vi "Get Devices List.vi"(0 "SLSC Interface in":refnum<class "SLSC Interface.lvclass">, 11 "error in (no error)":errorcluster) -> (4 "SLSC Interface out":refnum<class "SLSC Interface.lvclass">, 8 "Sys.Devices":refnum<k21>[](array[refnum]), 15 "error out":errorcluster)   [LabVIEW 2015, in "SLSC Interface.lvclass"]
uses:
  SLSC Interface.lvclass
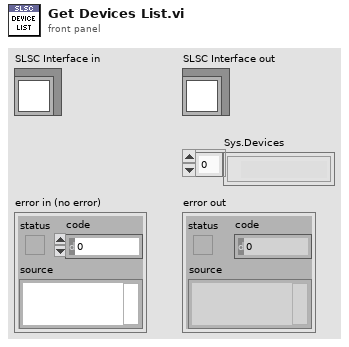
[diagram p1: front panel]
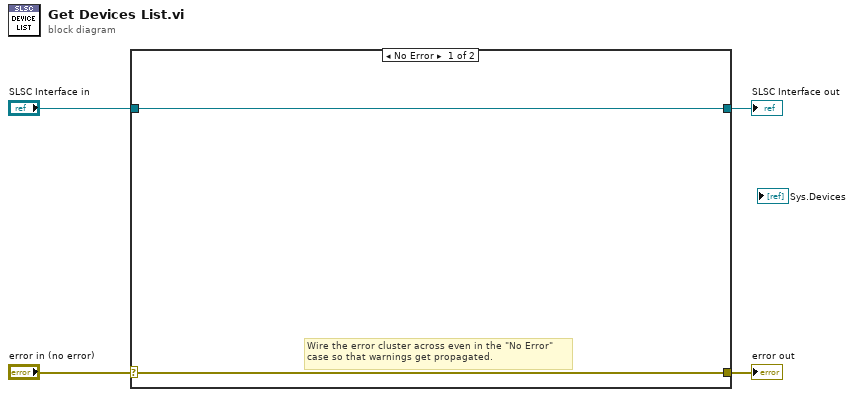
[diagram p0: block diagram]
diagram:
  n1 = case shown="No Error" "error in (no error)" {
    selector: "error in (no error)" -> [w5 w8]
    tunnel: [w5 w8] -> w3
    tunnel: [w6 w7] -> w1
    tunnel: "SLSC Interface in" -> [w6 w7]
    frame No Error {
      # "Wire the error cluster across even in the \"No Error\"\ncase so that warnings get propagated."
    }
    frame Error {
    }
  }
  "error out" <- w3
  "SLSC Interface out" <- w1
